vi "Ajustar_Escala_Senal.vi"(2 "Data_Canal_2":dbl, 3 "Data_Canal_1":dbl, 4 "Escala":dbl, 5 "Tipo_Canal":bool) -> (0 "Data_Canal_2":dbl, 1 "Data_Canal_1":dbl)   [LabVIEW 2023]
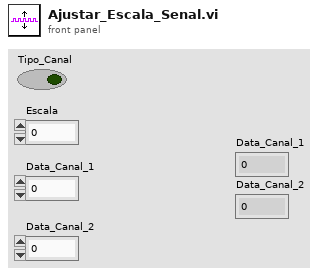
[diagram p1: front panel]
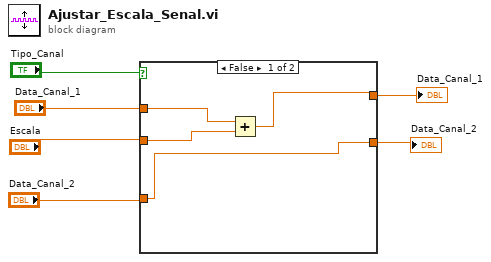
[diagram p0: block diagram]
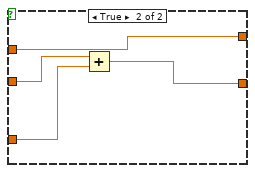
[diagram p2: hidden frame]
diagram:
  n1 = case shown="False" "Tipo_Canal" {
    tunnel: "Data_Canal_1" -> [w10 w13]
    tunnel: "Data_Canal_2" -> [w7 w11]
    tunnel: "Escala" -> [w9 w12]
    tunnel: [w7 w14] -> w1
    tunnel: [w8 w13] -> w2
    frame False {
      n2 = Add(x=w10, y=w9) -> (x+y=w8:dbl)
    }
    frame True {
      n3 = Add(x=w12, y=w11) -> (x+y=w14:dbl)
    }
  }
  "Data_Canal_1" <- w2
  "Data_Canal_2" <- w1
